vi "参数设置.vi"(11 "IN SRTING":string) -> (3 "pra out":string)   [LabVIEW 2011]
panel:
  in  "动作:":T1=5 items=["等待时间", "Y轴向后移动", "Y轴向前移动", "X轴向后移动", "X轴向前移动", "X向前Y向后移动", "Y向前X向后移动", "XY向前移动", "XY向后移动", ""]
  in  "返回":bool
  in  "保存":bool
  in  "删除":bool
  in  "参数名:":string(combo)
  in  "动态编程":i32(listbox)
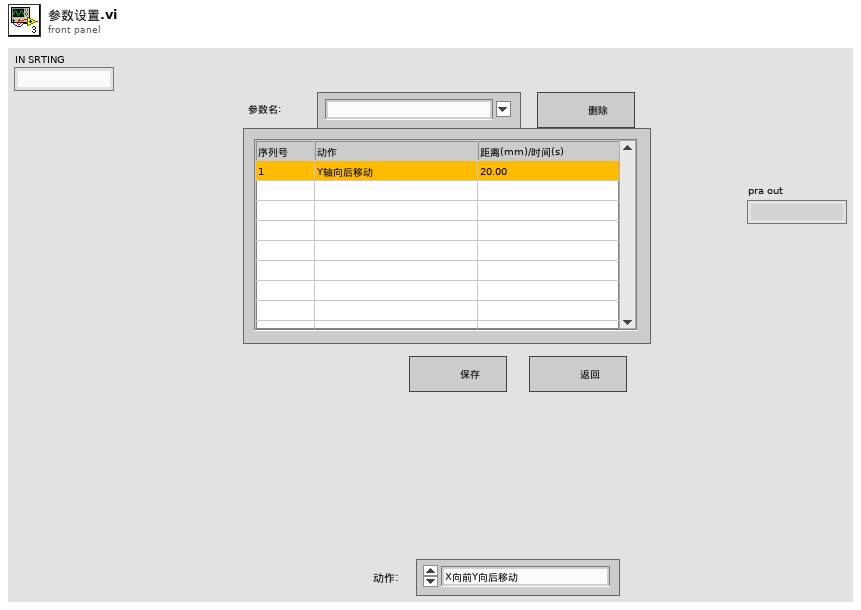
[diagram p1: front panel]
types:
  T1 = typedef "动作选项.ctl" = u16
  T2 = enum16{"open", "replace", "create", "open or create", "replace or create", "replace or create with confirmation"}
  T3 = typedef "动作机.ctl" = cluster{"动作:":T1, "参数：":dbl}
  T4 = typedef "LVPoint32TypeDef.ctl" = cluster{"Horizontal":i32, "Vertical":i32}
  T5 = typedef "LVRowAndColumnTypeDef.ctl" = cluster{"Row":i32, "Column":i32}
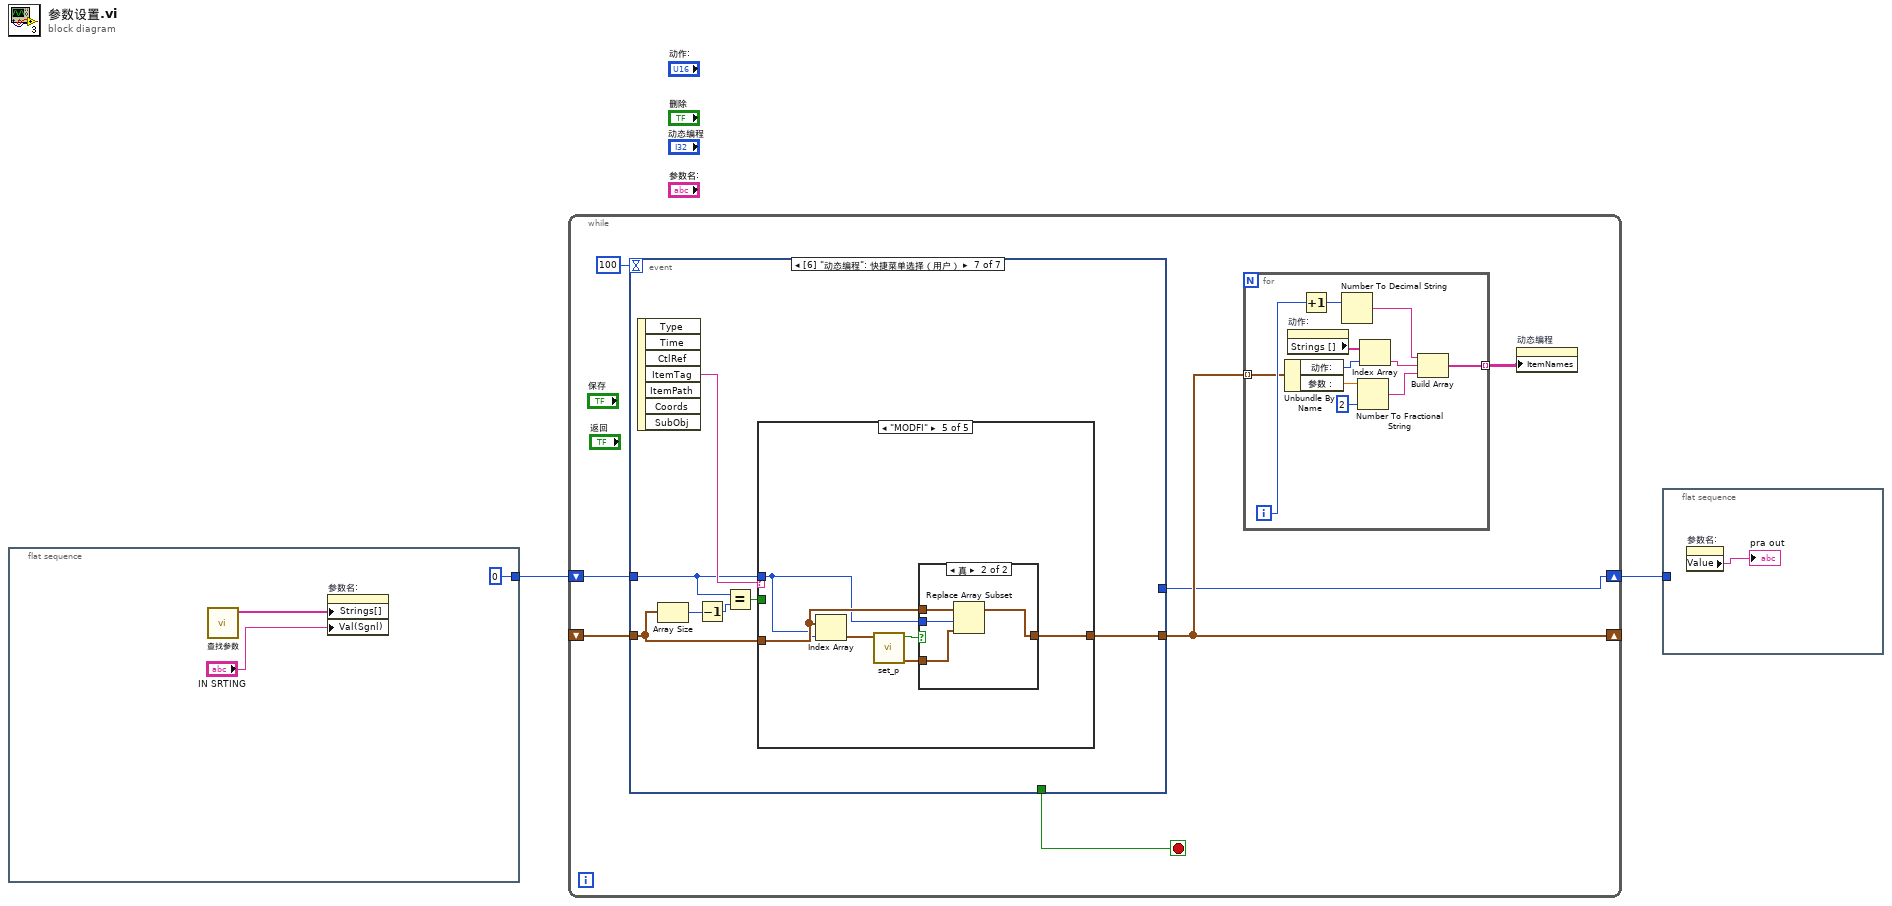
[diagram p0: block diagram]
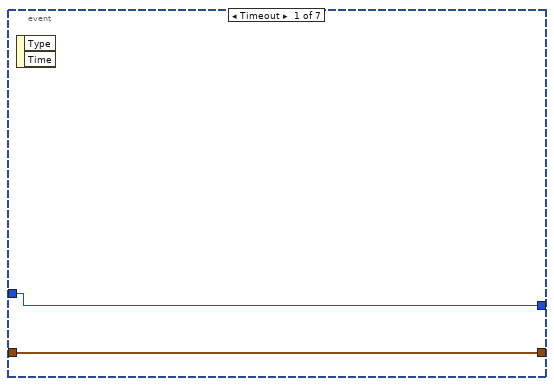
[diagram p2: hidden frame]
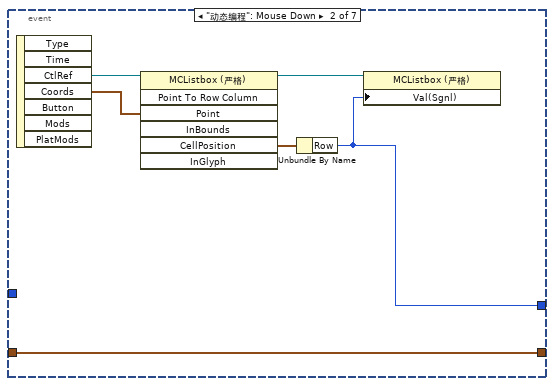
[diagram p3: hidden frame]
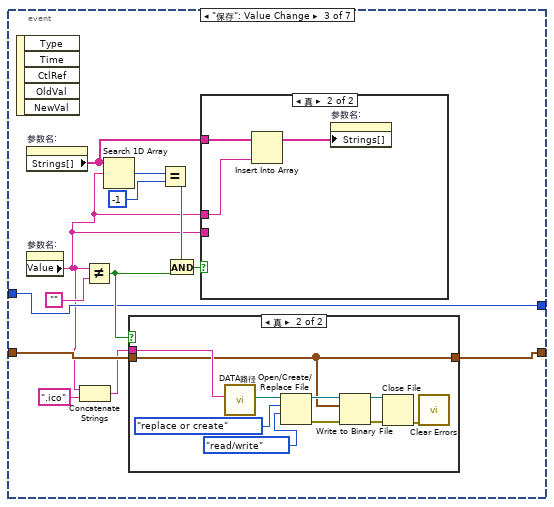
[diagram p4: hidden frame]
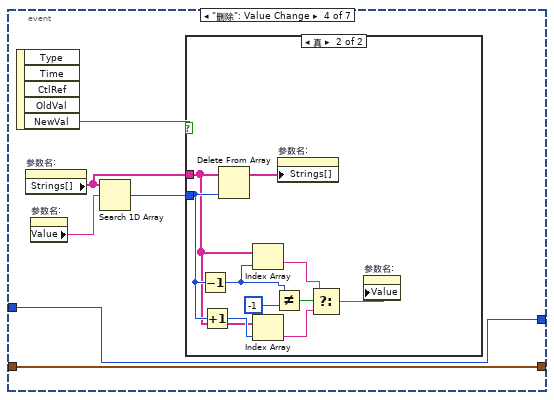
[diagram p7: hidden frame]
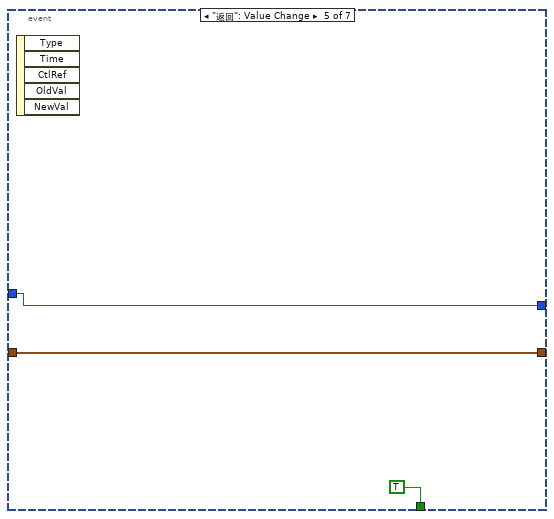
[diagram p9: hidden frame]
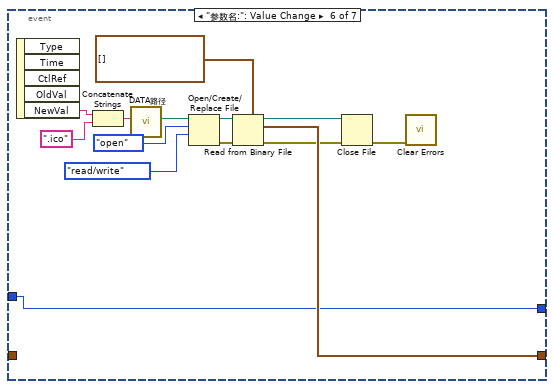
[diagram p10: hidden frame]
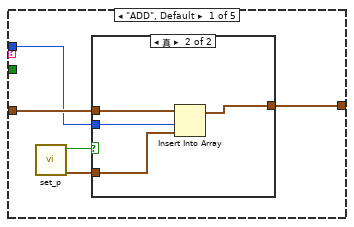
[diagram p11: hidden frame]
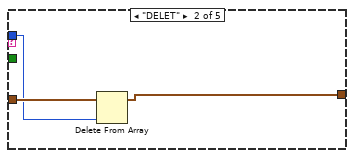
[diagram p13: hidden frame]
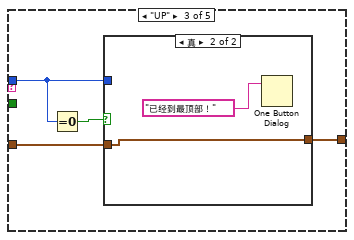
[diagram p14: hidden frame]
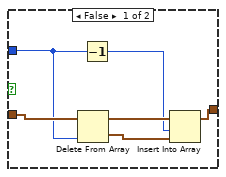
[diagram p15: hidden frame]
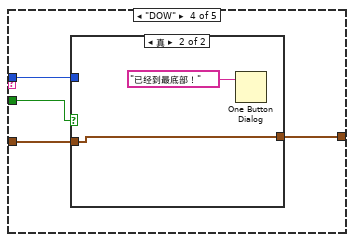
[diagram p16: hidden frame]
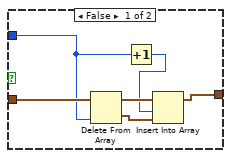
[diagram p17: hidden frame]
diagram:
  n1 = flat-sequence {
    tunnel: [0] -> w2
    frame #0 {
      n2 = call "查找参数.vi"() -> ("par name"=w5:string[])  [unwired: 11 in]
      n3 = property on="参数名:" class="CmbBox"("Strings[]"=w5, "Val(Sgnl)"="IN SRTING") -> ()  [unwired: 2 in, 2 out]
    }
  }
  n4 = while {
    shift-right: [w9] -> _
    shift-left: _ -> [w10]
    shift-right: [w6] -> w1
    shift-left: w2 -> [w7]
    stop <- w11 stop-if-true
    n5 = event shown="[6] \"动态编程\": 快捷菜单选择（用户）" {
      selector: _ -> [_ _ _ _ _ _ _]
      dyn-events: _ -> [_ _ _ _ _ _ _]
      timeout: 100 -> [_ _ _ _ _ _ _]
      tunnel: [_ _ _ _ TRUE _ _] -> w11
      tunnel: w10 -> [w25 w29 w37 w60 w76 _ w96]
      tunnel: [w25 w29 w36 w60 w76 w85 w97] -> w9
      tunnel: w7 -> [w24 _ w35 w59 w75 w81 w93]
      tunnel: [w24 w26 w35 w59 w75 w81 _] -> w6
      event Timeout {
        n6 = event-data() -> ()  [unwired: 1 in, 2 out]
      }
      event "动态编程": Mouse Down {
        n7 = event-data() -> ("CtlRef"=w28:refnum<vi>, "Coords"=w31:T4)  [unwired: 1 in, 5 out]
        n8 = invoke class="MCListbox (严格)" method="Point To Row Column"(reference=w28, "Point"=w31) -> (reference out=w27:refnum<vi>, "CellPosition"=w30:T5)  [unwired: 5 in, 5 out]
        n9 = Unbundle By Name(w30) -> ("Row"=w26:i32)
        n10 = property class="MCListbox (严格)"(reference=w27, "Val(Sgnl)"=w26) -> ()  [unwired: 1 in, 2 out]
      }
      event "保存": Value Change {
        n11 = event-data() -> ()  [unwired: 1 in, 5 out]
        n12 = property on="参数名:" class="CmbBox"() -> ("Strings[]"=w41:string[])  [unwired: 2 in, 2 out]
        n13 = property on="参数名:" class="CmbBox"() -> ("Value"=w34:string)  [unwired: 2 in, 2 out]
        n14 = Concatenate Strings(w34, ".ico" ("字符串")) -> (w32:string)
        n15 = Not Equal?(x=w34, y="") -> (x != y?=w38:bool)
        n16 = Search 1D Array(1D array=w41, element=w34) -> (index of element=w43:i32)  [unwired: 1 in]
        n17 = case shown="真" w38 {
          tunnel: w32 -> [_ w55]
          tunnel: w37 -> [w45 w46]
          tunnel: [w45 w46] -> w36
          frame False {
          }
          frame True {
            n18 = call "DATA路径.vi"("文件名"=w55) -> ("DATA路径"=w54:path)  [unwired: 10 in]
            n19 = Open/Create/Replace File(file path (use dialog)=w54, operation (0:open)=T2."replace or create" ("操作(0:open)"), access (0:read/write)=enum16{"read/write", "read-only", "write-only"}."read/write" ("权限(0:read/write)")) -> (refnum out=w51:refnum<file>, error out=w50:errorcluster)  [unwired: 3 in, 1 out]
            n20 = Write to Binary File(file (use dialog)=w51, data=w46, error in=w50) -> (refnum out=w49:refnum<file>, error out=w48:errorcluster)  [unwired: 3 in, 1 out]
            n21 = Close File(refnum=w49, error in=w48) -> (error out=w47:errorcluster)  [unwired: 1 out]
            n22 = call <vilib>:"Clear Errors.vi"("error in (no error)"=w47) -> ()  [unwired: 6 in, 1 out]
          }
        }
        n23 = Equal?(x=w43, y=-1) -> (x = y?=w39:bool)
        n24 = And(x=w39, y=w38) -> (x .and. y?=w40:bool)
        n25 = case shown="真" w40 {
          tunnel: w34 -> [_ _]
          tunnel: w41 -> [_ w58]
          tunnel: w34 -> [_ w57]
          frame False {
          }
          frame True {
            n26 = Insert Into Array(array=w58, new element=w57) -> (w56:string[])  [unwired: 1 in]
            n27 = property on="参数名:" class="CmbBox"("Strings[]"=w56) -> ()  [unwired: 2 in, 2 out]
          }
        }
      }
      event "删除": Value Change {
        n28 = event-data() -> ("NewVal"=w64:bool)  [unwired: 1 in, 4 out]
        n29 = property on="参数名:" class="CmbBox"() -> ("Strings[]"=w62:string[])  [unwired: 2 in, 2 out]
        n30 = property on="参数名:" class="CmbBox"() -> ("Value"=w63:string)  [unwired: 2 in, 2 out]
        n31 = Search 1D Array(1D array=w62, element=w63) -> (index of element=w61:i32)  [unwired: 1 in]
        n32 = case shown="真" w64 {
          tunnel: w61 -> [_ w73]
          tunnel: w62 -> [_ w69]
          frame False {
          }
          frame True {
            n33 = Decrement(x=w73) -> (x-1=w71:i32)
            n34 = Increment(x=w73) -> (x+1=w72:i32)
            n35 = Delete From Array(array=w69, index=w73) -> (array with subset deleted=w74:string[])  [unwired: 1 in, 1 out]
            n36 = Index Array(array=w69, index=w71) -> (element=w67:string)
            n37 = Index Array(array=w69, index=w72) -> (element=w66:string)
            n38 = Not Equal?(x=w71, y=-1) -> (x != y?=w68:bool)
            n39 = property on="参数名:" class="CmbBox"("Strings[]"=w74) -> ()  [unwired: 2 in, 2 out]
            n40 = Select(t=w67, s=w68, f=w66) -> (s? t:f=w65:string)
            n41 = property on="参数名:" class="CmbBox"("Value"=w65) -> ()  [unwired: 2 in, 2 out]
          }
        }
      }
      event "返回": Value Change {
        n42 = event-data() -> ()  [unwired: 1 in, 5 out]
      }
      event "参数名:": Value Change {
        n43 = event-data() -> ("NewVal"=w80:string)  [unwired: 1 in, 4 out]
        n44 = Concatenate Strings(w80, ".ico" ("字符串")) -> (w78:string)
        n45 = call "DATA路径.vi"("文件名"=w78) -> ("DATA路径"=w91:path)  [unwired: 10 in]
        n46 = Open/Create/Replace File(file path (use dialog)=w91, operation (0:open)=T2."open" ("操作(0:open)"), access (0:read/write)=enum16{"read/write", "read-only", "write-only"}."read/write" ("权限(0:read/write)")) -> (refnum out=w88:refnum<file>, error out=w87:errorcluster)  [unwired: 3 in, 1 out]
        n47 = Read from Binary File(5:T3[] [], 8:w87, 11:w88) -> (0:w84:errorcluster, 2:w85:T3[], 3:w83:refnum<file>)  [unwired: 3 in, 1 out]
        n48 = Close File(refnum=w83, error in=w84) -> (error out=w82:errorcluster)  [unwired: 1 out]
        n49 = call <vilib>:"Clear Errors.vi"("error in (no error)"=w82) -> ()  [unwired: 6 in, 1 out]
      }
      event "动态编程": Shortcut Menu Selection (User) {
        n50 = event-data() -> ("ItemTag"=w98:string)  [unwired: 1 in, 6 out]
        n51 = Array Size(array=w96) -> (size(s)=w95:i32)
        n52 = Decrement(x=w95) -> (x-1=w94:i32)
        n53 = Equal?(x=w93, y=w94) -> (x = y?=w92:bool)
        n54 = case shown="\"MODFI\"" w98 {
          tunnel: w96 -> [w101 w111 w115 w127 w140]
          tunnel: [w100 w109 w114 w125 w136] -> w97
          tunnel: w93 -> [w99 w110 w113 w126 w139]
          tunnel: w92 -> [_ _ _ w124 _]
          frame "ADD", Default {
            n55 = call "set_p.vi"() -> ("动作机 OUT"=w102:T3, "OK"=w103:bool)  [unwired: 10 in]
            n56 = case shown="真" w103 {
              tunnel: w102 -> [_ w107]
              tunnel: w101 -> [w104 w108]
              tunnel: [w104 w106] -> w100
              tunnel: w99 -> [_ w105]
              frame False {
              }
              frame True {
                n57 = Insert Into Array(array=w108, index=w105, new element=w107) -> (w106:T3[])
              }
            }
          }
          frame "DELET" {
            n58 = Delete From Array(array=w111, index=w110) -> (array with subset deleted=w109:T3[])  [unwired: 1 in, 1 out]
          }
          frame "UP" {
            n59 = Equal To 0?(x=w113) -> (x = 0?=w112:bool)
            n60 = case shown="真" w112 {
              tunnel: w115 -> [w121 w123]
              tunnel: [w117 w123] -> w114
              tunnel: w113 -> [w116 _]
              frame False {
                n61 = Delete From Array(array=w121, index=w116) -> (deleted portion=w118:T3, array with subset deleted=w120:T3[])  [unwired: 1 in]
                n62 = Decrement(x=w116) -> (x-1=w119:i32)
                n63 = Insert Into Array(array=w120, index=w119, new element=w118) -> (w117:T3[])
              }
              frame True {
                n64 = One Button Dialog(message="已经到最顶部！" ("消息")) -> ()  [unwired: 1 in, 1 out]
              }
            }
          }
          frame "DOW" {
            n65 = case shown="真" w124 {
              tunnel: w127 -> [w133 w135]
              tunnel: w126 -> [w131 _]
              tunnel: [w128 w135] -> w125
              frame False {
                n66 = Delete From Array(array=w133, index=w131) -> (deleted portion=w129:T3, array with subset deleted=w132:T3[])  [unwired: 1 in]
                n67 = Increment(x=w131) -> (x+1=w130:i32)
                n68 = Insert Into Array(array=w132, index=w130, new element=w129) -> (w128:T3[])
              }
              frame True {
                n69 = One Button Dialog(message="已经到最底部！" ("消息")) -> ()  [unwired: 1 in, 1 out]
              }
            }
          }
          frame "MODFI" {
            n70 = Index Array(array=w140, index=w139) -> (element=w141:T3)
            n71 = call "set_p.vi"("动作机 IN"=w141) -> ("动作机 OUT"=w138:T3, "OK"=w137:bool)  [unwired: 9 in]
            n72 = case shown="真" w137 {
              tunnel: w140 -> [w142 w146]
              tunnel: w139 -> [_ w145]
              tunnel: w138 -> [_ w144]
              tunnel: [w142 w143] -> w136
              frame False {
              }
              frame True {
                n73 = Replace Array Subset(array=w146, new element=w144, index=w145) -> (w143:T3[])
              }
            }
          }
        }
      }
    }
    n74 = for {
      tunnel: w9 -> [w22] mode=indexing
      tunnel: [w13] -> w8 mode=indexing
      i -> [w23]
      n75 = Unbundle By Name(w22) -> ("动作:"=w17:T1, "参数："=w21:dbl)
      n76 = property on="动作:" class="Ring (严格)"() -> ("Strings []"=w18:string[])  [unwired: 2 in, 2 out]
      n77 = Increment(x=w23) -> (x+1=w15:i32)
      n78 = Number To Decimal String(number=w15) -> (decimal integer string=w14:string)  [unwired: 1 in]
      n79 = Number To Fractional String(number=w21, precision (6)=i16 2 ("精度(6)")) -> (F-format string=w19:string)  [unwired: 2 in]
      n80 = Index Array(array=w18, index=w17) -> (element=w16:string)
      n81 = Build Array(w14, w16, w19) -> (w13:string[])
    }
    n82 = property on="动态编程" class="MCListbox (严格)"("ItemNames"=w8) -> ()  [unwired: 2 in, 2 out]
  }
  n83 = flat-sequence {
    tunnel: w1 -> [_]
    frame #0 {
      n84 = property on="参数名:" class="CmbBox"() -> ("Value"=→"pra out":string)  [unwired: 2 in, 2 out]
    }
  }
